vi "ParkCost.vi"(5 "Date/time":string, 6 "OldVal":bool, 7 "Log in":string, 8 "NewVal":bool, 9 "Seconds":dbl, 10 "Bay index":i32, 11 "S array":refnum<vi>[](array[refnum])) -> (1 "Log out":string, 3 "ParkCost":string)   [LabVIEW 2023]
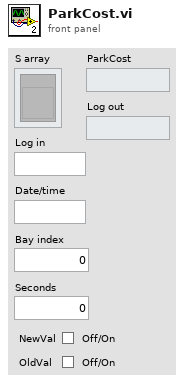
[diagram p1: front panel]
types:
  T1 = cluster{"Time String":string, "h":i32, "m":i32, ">30m":bool, "s":i32, "Cost":dbl}
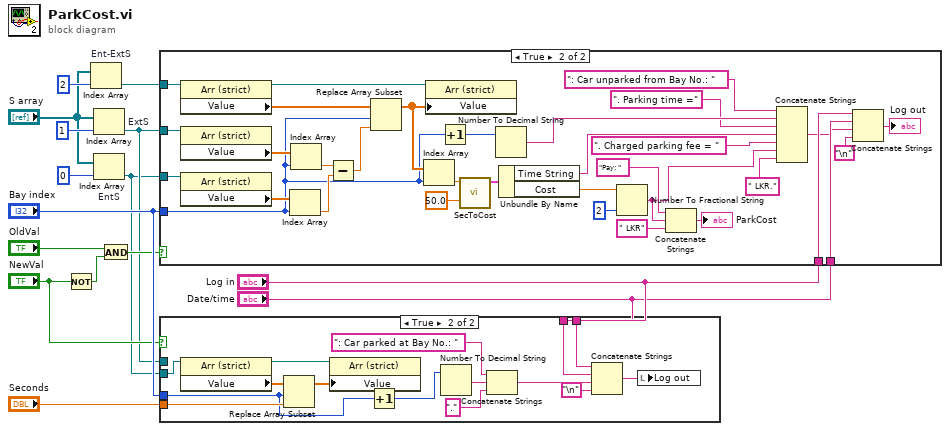
[diagram p0: block diagram]
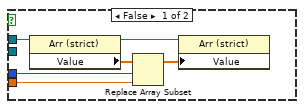
[diagram p3: hidden frame]
diagram:
  n1 = Not(x="NewVal") -> (.not. x?=w13:bool)
  n2 = Index Array "Ent-ExtS"(array="S array", index=2) -> (element=w4:refnum<vi>)
  n3 = Index Array "ExtS"(array="S array", index=1) -> (element=w5:refnum<vi>)
  n4 = Index Array "EntS"(array="S array", index=0) -> (element=w3:refnum<vi>)
  n5 = And(x="OldVal", y=w13) -> (x .and. y?=w14:bool)
  n6 = case shown="True" w14 {
    tunnel: "Bay index" -> [_ w26]
    tunnel: w5 -> [_ w35]
    tunnel: w3 -> [_ w34]
    tunnel: w4 -> [_ w33]
    tunnel: "Log in" -> [_ w23]
    tunnel: "Date/time" -> [_ w22]
    frame False {
    }
    frame True {
      n7 = property class="Arr (strict)"(reference=w33) -> (reference out=w32:refnum<vi>, "Value"=w46:dbl[])  [unwired: 1 in, 1 out]
      n8 = property class="Arr (strict)"(reference=w35) -> ("Value"=w48:dbl[])  [unwired: 1 in, 2 out]
      n9 = property class="Arr (strict)"(reference=w34) -> ("Value"=w47:dbl[])  [unwired: 1 in, 2 out]
      n10 = Index Array(array=w47, index=w26) -> (element=w44:dbl)
      n11 = Index Array(array=w48, index=w26) -> (element=w45:dbl)
      n12 = Subtract(x=w45, y=w44) -> (x-y=w43:dbl)
      n13 = Replace Array Subset(array=w46, new element=w43, index=w26) -> (w42:dbl[])
      n14 = Index Array(array=w42, index=w26) -> (element=w41:dbl)
      n15 = property class="Arr (strict)"(reference=w32, "Value"=w42) -> ()  [unwired: 1 in, 2 out]
      n16 = Increment(x=w26) -> (x+1=w24:i32)
      n17 = call "SecToCost.vi"("Rate"=50.0, "Seconds"=w41) -> ("StoCcluster"=w39:T1)  [unwired: 9 in]
      n18 = Number To Decimal String(number=w24) -> (decimal integer string=w25:string)  [unwired: 1 in]
      n19 = Unbundle By Name(w39) -> ("Time String"=w18:string, "Cost"=w37:dbl)
      n20 = Number To Fractional String(number=w37, precision (6)=i16 2) -> (F-format string=w16:string)  [unwired: 2 in]
      n21 = Concatenate Strings("Pay: " ("string"), w16, " LKR" ("string")) -> (→"ParkCost":string)
      n22 = Concatenate Strings(": Car unparked from Bay No.: " ("string"), w25, ". Parking time =" ("string"), w18, ". Charged parking fee = " ("string"), w16, " LKR." ("string")) -> (w20:string)
      n23 = Concatenate Strings(w23, w22, w20, "\n") -> (→"Log out":string)
    }
  }
  n24 = case shown="True" "NewVal" {
    tunnel: "Seconds" -> [w52 w68]
    tunnel: "Bay index" -> [w51 w61]
    tunnel: w5 -> [w50 _]
    tunnel: w3 -> [_ w66]
    tunnel: "Log in" -> [_ w56]
    tunnel: "Date/time" -> [_ w55]
    frame False {
      n25 = property class="Arr (strict)"(reference=w50) -> (reference out=w49:refnum<vi>, "Value"=w54:dbl[])  [unwired: 1 in, 1 out]
      n26 = Replace Array Subset(array=w54, new element=w52, index=w51) -> (w53:dbl[])
      n27 = property class="Arr (strict)"(reference=w49, "Value"=w53) -> ()  [unwired: 1 in, 2 out]
    }
    frame True {
      n28 = property class="Arr (strict)"(reference=w66) -> (reference out=w65:refnum<vi>, "Value"=w69:dbl[])  [unwired: 1 in, 1 out]
      n29 = Replace Array Subset(array=w69, new element=w68, index=w61) -> (w67:dbl[])
      n30 = property class="Arr (strict)"(reference=w65, "Value"=w67) -> ()  [unwired: 1 in, 2 out]
      n31 = Increment(x=w61) -> (x+1=w60:i32)
      n32 = Number To Decimal String(number=w60) -> (decimal integer string=w63:string)  [unwired: 1 in]
      n33 = Concatenate Strings(": Car parked at Bay No.: " ("string"), w63, "." ("string")) -> (w58:string)
      n34 = Concatenate Strings(w56, w55, w58, "\n") -> (w57:string)
      n35 = local write "Log out"(w57) -> ()
    }
  }
